vi "toJSON.vi"(8 "error in (no error)":errorcluster, 11 "tBSONElement in":refnum<class "tBSONElement.lvclass">) -> (0 "error out":errorcluster, 2 "JSON":string, 3 "tBSONElement out":refnum<class "tBSONElement.lvclass">)   [LabVIEW 2013, in "BSON.lvlib" / "tBSONElement.lvclass"]
doc: "Converts a BSON element into JSON text representing the element."
uses:
  tBSONElement.lvclass
  getName.vi
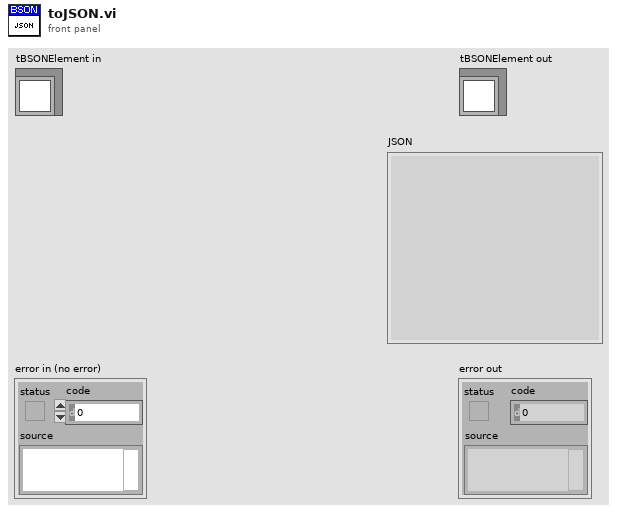
[diagram p1: front panel]
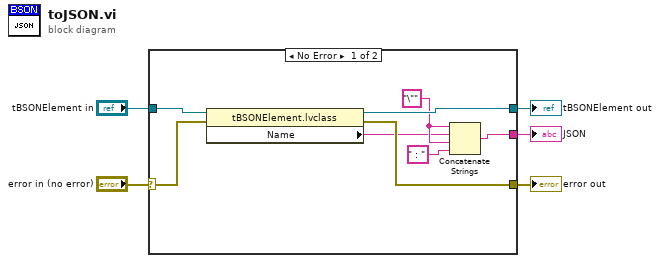
[diagram p0: block diagram]
diagram:
  n1 = case shown="No Error" "error in (no error)" {
    selector: "error in (no error)" -> [w12 w15]
    tunnel: [w10 w15] -> w4
    tunnel: [w11 w14] -> w2
    tunnel: "tBSONElement in" -> [w13 w14]
    tunnel: [w6 _] -> w1
    frame No Error {
      w9 = "\"" ("string")
      n2 = property class="tBSONElement.lvclass"(reference=w13, error in=w12) -> (reference out=w11:refnum<class "tBSONElement.lvclass">, error out=w10:errorcluster, "Name"=w8:string)
      n3 = Concatenate Strings(w9, w8, w9, " : " ("string")) -> (w6:string)
    }
    frame Error {
    }
  }
  "error out" <- w4
  "tBSONElement out" <- w2
  "JSON" <- w1
